vi "YokoGS200 VisaRW.vi"(0 "VISA Rsrc":refnum<visa-resource-name>="SR530", 2 "EOS (Aucun)":string, 3 "Délais (0 ms)":u32, 5 "ChaineCom":string caption="Chaîne de commande", 7 "Nbcomm":i32=1 caption="Nombre de \nCommandes", 9 "Nbcaract":u32=100 caption="Nombre de \ncaractères à lire", 11 "error in (no error)":errorcluster, 12 "Lecture?(T)":bool=TRUE, 13 "Poll?(F)":bool) -> (4 "VISA Rsrc Out":refnum<visa-resource-name>="GPIB0::12::INSTR", 6 "ChaineRep":string caption="Chaîne de réponse", 8 "octet d'état":u16, 14 "Count out":u32=44 caption="Nombre de caractères lus", 15 "error out":errorcluster)   [LabVIEW 2012]
doc: "Ce VI envoie des commande d'écriture et de lecture VISA à l'appareil GPIB. Il permet de ne pas séparer un question de sa réponse. Pour que cela fonctionne toute lecture d'un instrument doit se faire par ce VI."
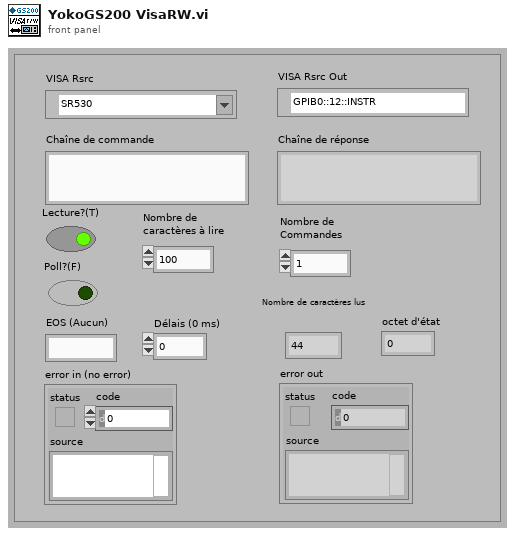
[diagram p1: front panel]
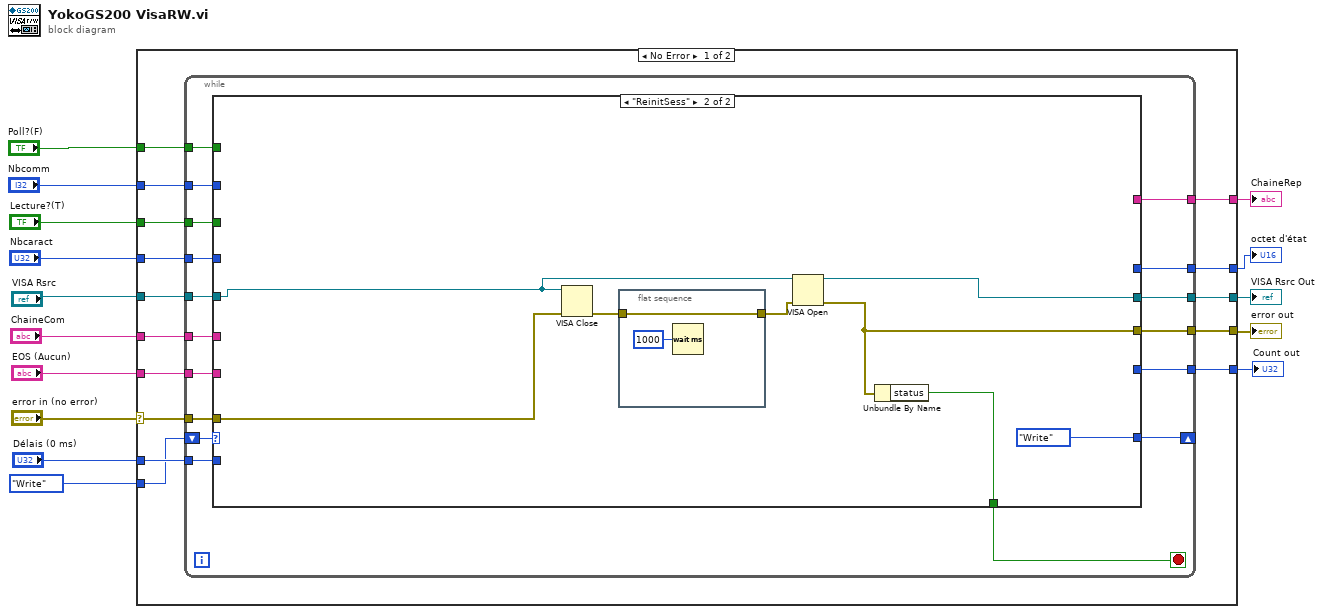
[diagram p0: block diagram]
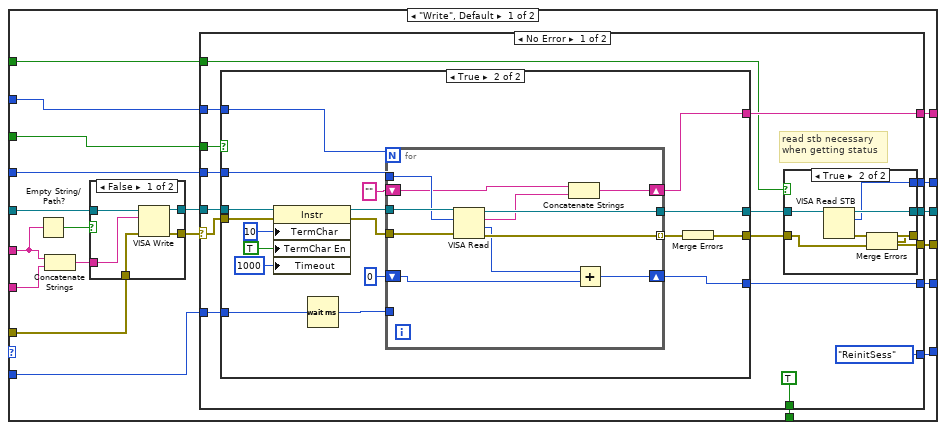
[diagram p2: hidden frame]
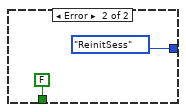
[diagram p5: hidden frame]
diagram:
  n1 = case shown="No Error" "error in (no error)" {
    selector: "error in (no error)" -> [w28 w143]
    tunnel: "VISA Rsrc" -> [w29 w142]
    tunnel: [w19 w142] -> w8
    tunnel: "ChaineCom" -> [w21 _]
    tunnel: "EOS (Aucun)" -> [w30 _]
    tunnel: "Délais (0 ms)" -> [w27 _]
    tunnel: "Nbcaract" -> [w26 _]
    tunnel: "Lecture?(T)" -> [w25 _]
    tunnel: [w18 w143] -> w10
    tunnel: "Nbcomm" -> [w22 _]
    tunnel: [w24 _] -> w6
    tunnel: [w23 _] -> w5
    tunnel: "Poll?(F)" -> [w20 _]
    tunnel: [w17 _] -> w2
    tunnel: enum16{"Write", "ReinitSess"}."Write" -> [w16 _]
    frame No Error {
      n2 = while {
        tunnel: w30 -> [w47]
        tunnel: w29 -> [w46]
        tunnel: w28 -> [w45]
        tunnel: w27 -> [w44]
        tunnel: w26 -> [w43]
        tunnel: w25 -> [w42]
        tunnel: [w41] -> w24
        tunnel: [w40] -> w23
        tunnel: w22 -> [w39]
        tunnel: w21 -> [w38]
        tunnel: w20 -> [w37]
        tunnel: [w36] -> w19
        tunnel: [w35] -> w18
        tunnel: [w34] -> w17
        shift-right: [w32] -> _
        shift-left: w16 -> [w33]
        stop <- w31 stop-if-true
        n3 = case shown="\"ReinitSess\"" w33 {
          tunnel: w47 -> [w67 _]
          tunnel: w46 -> [w65 w138]
          tunnel: w45 -> [w64 w139]
          tunnel: w44 -> [w62 _]
          tunnel: w43 -> [w61 _]
          tunnel: w42 -> [w60 _]
          tunnel: [w59 _] -> w41
          tunnel: [w58 _] -> w40
          tunnel: w39 -> [w57 _]
          tunnel: w38 -> [w56 _]
          tunnel: w37 -> [w54 _]
          tunnel: [w53 w137] -> w36
          tunnel: [w52 w135] -> w35
          tunnel: [w51 _] -> w34
          tunnel: [w50 enum16{"Write", "ReinitSess"}."Write"] -> w32
          tunnel: [w48 w134] -> w31
          frame "Write", Default {
            n4 = Empty String/Path?(string/path=w56) -> (empty?=w55:bool)
            n5 = Concatenate Strings(w56, w67) -> (w66:string)
            n6 = case shown="False" w55 {
              tunnel: w66 -> [w129 _]
              tunnel: w65 -> [w128 w131]
              tunnel: w64 -> [w127 w130]
              tunnel: [w126 w131] -> w63
              tunnel: [w125 w130] -> w49
              frame False {
                n7 = VISA Write(VISA resource name=w128, write buffer=w129, error in (no error)=w127) -> (VISA resource name out=w126:refnum<visa-resource-name>, error out=w125:errorcluster)  [unwired: 1 out]
              }
              frame True {
              }
            }
            n8 = case shown="No Error" w49 {
              selector: w49 -> [w69 _]
              tunnel: w63 -> [w83 _]
              tunnel: w62 -> [w82 _]
              tunnel: w61 -> [w81 _]
              tunnel: w60 -> [w80 _]
              tunnel: [w79 _] -> w59
              tunnel: [w78 _] -> w58
              tunnel: w57 -> [w77 _]
              tunnel: w54 -> [w76 _]
              tunnel: [w73 _] -> w53
              tunnel: [w72 _] -> w52
              tunnel: [w71 _] -> w51
              tunnel: [enum16{"Write", "ReinitSess"}."ReinitSess" enum16{"Write", "ReinitSess"}."ReinitSess"] -> w50
              tunnel: [TRUE FALSE] -> w48
              frame No Error {
                # "read stb necessary\nwhen getting status"
                n9 = case shown="True" w80 {
                  tunnel: w83 -> [w93 w111]
                  tunnel: [w93 w95] -> w74
                  tunnel: w69 -> [w92 w100]
                  tunnel: [w92 w94] -> w75
                  tunnel: w81 -> [_ w109]
                  tunnel: w82 -> [_ w108]
                  tunnel: w77 -> [_ w102]
                  tunnel: [_ w104] -> w79
                  tunnel: [_ w103] -> w78
                  frame False {
                  }
                  frame True {
                    n10 = property class="Instr"(reference=w111, error in=w100, "TermChar"=u8 10 ("Message Based Settings:Termination Character"), "TermChar En"=TRUE ("Message Based Settings:Termination Character Enable"), "Timeout"=u32 1000 ("General Settings:Timeout Value")) -> (reference out=w101:refnum<visa-resource-name>, error out=w99:errorcluster)
                    n11 = Wait (ms)(milliseconds to wait=w108) -> (millisecond timer value=w107:u32)
                    n12 = for {
                      N: w102 -> [_]
                      tunnel: w101 -> [w122]
                      tunnel: [w121] -> w95
                      tunnel: w99 -> [w120]
                      tunnel: [w119] -> w110 mode=indexing
                      tunnel: w109 -> [w118]
                      tunnel: w107 -> [_]
                      shift-right: [w116] -> w104
                      shift-left: "" -> [w115]
                      shift-right: [w113] -> w103
                      shift-left: u32 0 -> [w112]
                      n13 = VISA Read(VISA resource name=w122, byte count=w118, error in (no error)=w120) -> (VISA resource name out=w121:refnum<visa-resource-name>, read buffer=w117:string, return count=w114:u32, error out=w119:errorcluster)
                      n14 = Concatenate Strings(w115, w117) -> (w116:string)
                      n15 = Add(x=w114, y=w112) -> (x+y=w113:u32)
                    }
                    n16 = Merge Errors(w110) -> (w94:errorcluster)
                  }
                }
                n17 = case shown="True" w76 {
                  tunnel: [w85 w91] -> w73
                  tunnel: [w84 w86] -> w72
                  tunnel: w75 -> [w84 w88]
                  tunnel: w74 -> [w85 w90]
                  tunnel: [_ w89] -> w71
                  frame False {
                  }
                  frame True {
                    n18 = VISA Read STB(11:w90) -> (0:w87:errorcluster, 2:w89:u16, 3:w91:refnum<visa-resource-name>)  [unwired: 1 in]
                    n19 = Merge Errors(w87, w88) -> (w86:errorcluster)
                  }
                }
              }
              frame Error {
              }
            }
          }
          frame "ReinitSess" {
            n20 = VISA Close(VISA resource name=w138, error in (no error)=w139) -> (error out=w132:errorcluster)
            n21 = flat-sequence {
              tunnel: [w140] -> w133
              tunnel: w132 -> [w140]
              frame #0 {
                n22 = Wait (ms)(milliseconds to wait=u32 1000) -> ()  [unwired: 1 out]
              }
            }
            n23 = VISA Open(error in (no error)=w133, VISA resource name=w138) -> (VISA resource name=w137:refnum<visa-resource-name>, error out=w135:errorcluster)  [unwired: 3 in]
            n24 = Unbundle By Name(w135) -> ("status"=w134:bool)
          }
        }
      }
    }
    frame Error {
    }
  }
  "error out" <- w10
  "VISA Rsrc Out" <- w8
  "ChaineRep" <- w6
  "Count out" <- w5
  "octet d'état" <- w2
